vi "RESTful INI Keyword ID CHAR.vi"() -> (3 "Keyword ID CHAR":string)   [LabVIEW 2020]
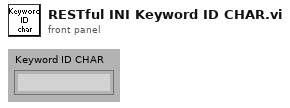
[diagram p1: front panel]
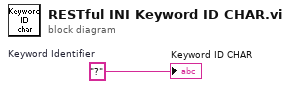
[diagram p0: block diagram]
diagram:
  w1 = "?"  # Keyword Identifier
  "Keyword ID CHAR" <- w1
